vi "readSettingsFile.vi"(8 "error in (no error)":errorcluster, 11 "Controller in":refnum<class "Controller.lvclass">) -> (0 "error out":errorcluster, 3 "Controller out":refnum<class "Controller.lvclass">)   [LabVIEW 2019, in "Controller.lvclass"]
uses:
  Controller.lvclass
  Controller.lvclass/Controller.ctl
  Axis/Axis.lvclass
  SMOs/Controller.LV/Controller.LV.lvclass
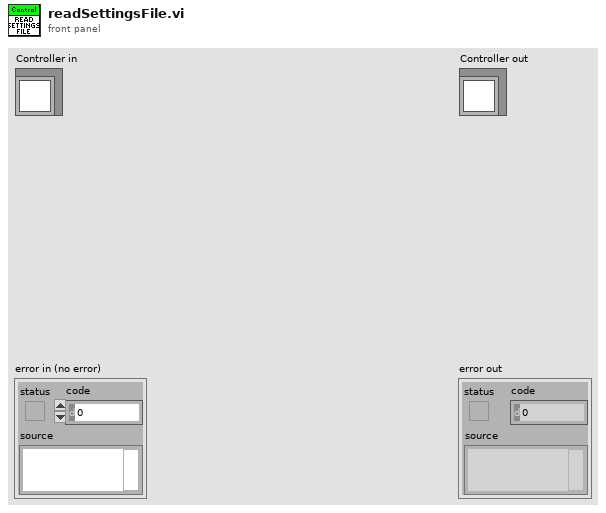
[diagram p1: front panel]
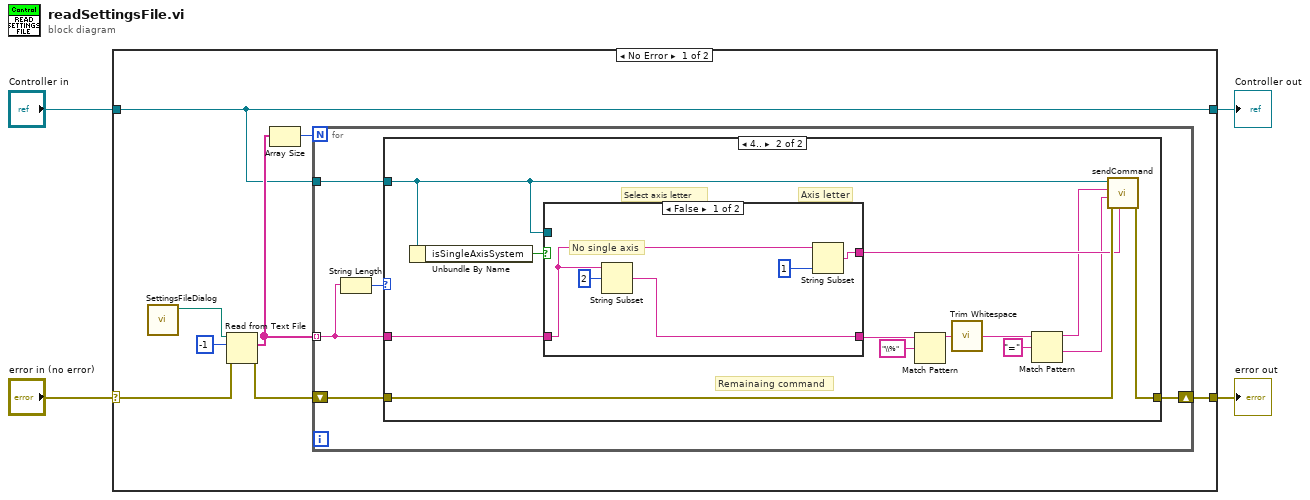
[diagram p0: block diagram]
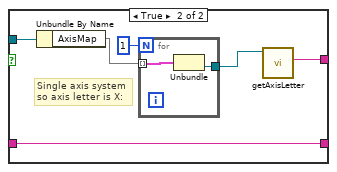
[diagram p3: hidden frame]
diagram:
  n1 = case shown="No Error" "error in (no error)" {
    selector: "error in (no error)" -> [w7 w46]
    tunnel: [w8 w46] -> w3
    tunnel: [w6 w45] -> w1
    tunnel: "Controller in" -> [w6 w45]
    frame No Error {
      n2 = call "SettingsFileDialog.vi"() -> ("selected path"=w5:path)  [unwired: 10 in, 1 out]
      n3 = Read from Text File(file (use dialog)=w5, count=-1, error in=w7) -> (text=w10:string[], error out=w9:errorcluster)  [unwired: 1 in, 2 out]
      n4 = Array Size(array=w10) -> (size(s)=w11:i32)
      n5 = for {
        N: w11 -> [_]
        tunnel: w10 -> [w16] mode=indexing
        shift-right: [w14] -> w8
        shift-left: w9 -> [w15]
        tunnel: w6 -> [w13]
        n6 = String Length(string=w16) -> (length=w17:i32)
        n7 = case shown="4.." w17 {
          tunnel: w16 -> [_ w30]
          tunnel: w15 -> [w18 w28]
          tunnel: [w18 w27] -> w14
          tunnel: w13 -> [_ w29]
          frame 0, Default {
          }
          frame 4.. {
            # "Remainaing command"
            # "Axis letter"
            # "Select axis letter"
            n8 = Unbundle By Name(w29) -> ("isSingleAxisSystem"=w31:bool)
            n9 = case shown="False" w31 {
              tunnel: w30 -> [w33 w42]
              tunnel: [w32 w42] -> w20
              tunnel: [w35 w40] -> w26
              tunnel: w29 -> [_ w41]
              frame False {
                # "No single axis"
                n10 = String Subset(string=w33, offset (0)=2) -> (substring=w32:string)  [unwired: 1 in]
                n11 = String Subset(string=w33, length (rest)=1) -> (substring=w35:string)  [unwired: 1 in]
              }
              frame True {
                # "Single axis system \nso axis letter is X:"
                n12 = Unbundle By Name(w41) -> ("AxisMap"=w37:map{string, refnum<class "Axis.lvclass">})
                n13 = for {
                  N: 1 -> [_]
                  tunnel: w37 -> [w44] mode=indexing
                  tunnel: [w43] -> w38
                  n14 = Unbundle(w44) -> ("Axis.lvclass"=w43:refnum<class "Axis.lvclass">)  [unwired: 1 out]
                }
                n15 = call-dynamic "getAxisLetter.vi"("Axis in"=w38) -> ("Axis Letter"=w40:string)  [unwired: 8 in, 2 out]
              }
            }
            n16 = Match Pattern(string=w20, regular expression="\\%") -> (before substring=w21:string)  [unwired: 1 in, 3 out]
            n17 = call <vilib>:"Trim Whitespace.vi"("string"=w21) -> ("trimmed string"=w19:string)  [unwired: 1 in]
            n18 = Match Pattern(string=w19, regular expression="=") -> (before substring=w24:string, after substring=w23:string)  [unwired: 1 in, 2 out]
            n19 = call-dynamic "sendCommand.vi"("Axis Letter"=w26, "error in (no error)"=w28, "Value"=w23, "Command"=w24, "Controller in"=w29) -> ("error out"=w27:errorcluster)  [unwired: 5 in, 1 out]
          }
        }
      }
    }
    frame Error {
    }
  }
  "error out" <- w3
  "Controller out" <- w1
